vi "Generate Archive Locations.vi"(8 "error in (no error)":errorcluster, 11 "Archivist In":refnum<class "Archivist.lvclass">) -> (0 "error out":errorcluster, 1 "Settings Paths":T1, 3 "Archivist Out":refnum<class "Archivist.lvclass">)   [LabVIEW 2019, in "Archivist.lvclass"]
uses:
  Archivist.lvclass
  Archivist.lvclass/Archivist.ctl
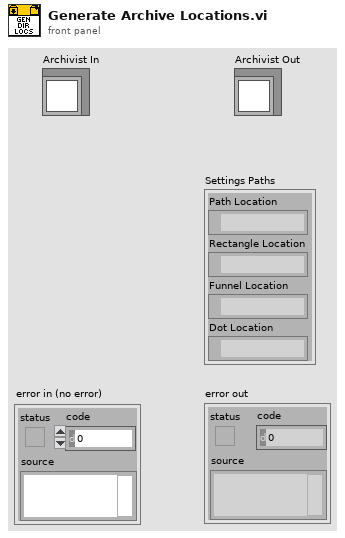
[diagram p1: front panel]
types:
  T1 = cluster{"Path Location":path, "Rectangle Location":path, "Funnel Location":path, "Dot Location":path}
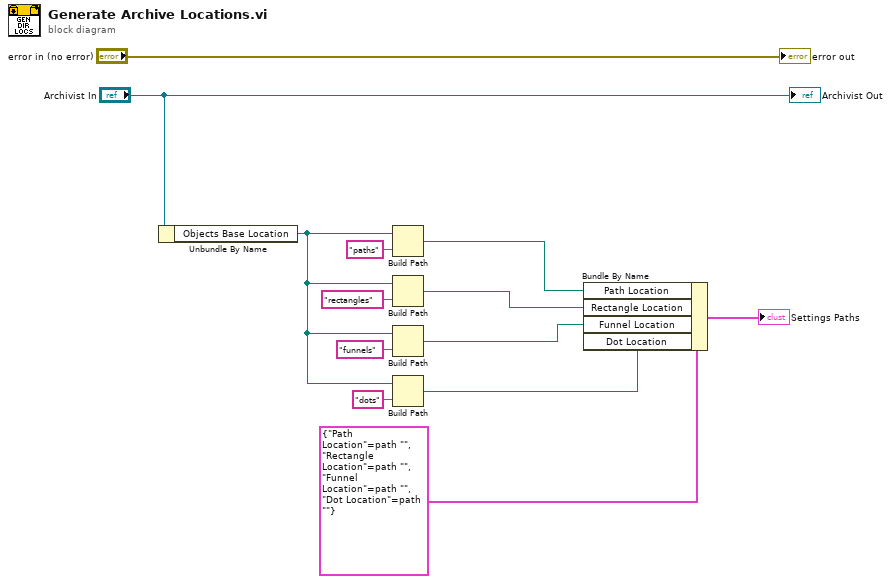
[diagram p0: block diagram]
diagram:
  n1 = Unbundle By Name("Archivist In") -> ("Objects Base Location"=w2:path)
  n2 = Build Path(base path=w2, name or relative path="paths") -> (appended path=w7:path)
  n3 = Build Path(base path=w2, name or relative path="rectangles") -> (appended path=w6:path)
  n4 = Build Path(base path=w2, name or relative path="funnels") -> (appended path=w5:path)
  n5 = Build Path(base path=w2, name or relative path="dots") -> (appended path=w4:path)
  n6 = Bundle By Name(cluster=T1 {"Path Location"=path "", "Rectangle Location"=path "", "Funnel Location"=path "", "Dot Location"=path ""}, "Path Location"=w7, "Rectangle Location"=w6, "Funnel Location"=w5, "Dot Location"=w4) -> (→"Settings Paths":T1)
  "error out" <- "error in (no error)"
  "Archivist Out" <- "Archivist In"
